vi "WriteCSV.vi"(9 "array":dbl[](array[numeric])=[1.12, 3.14, 0.0], 11 "file path (use dialog)":path=path "C:/Users/RoboIme/git/sslview/Util/Farias2.csv") -> ()   [LabVIEW 2018]
panel:
  out "refnum out":refnum<file>
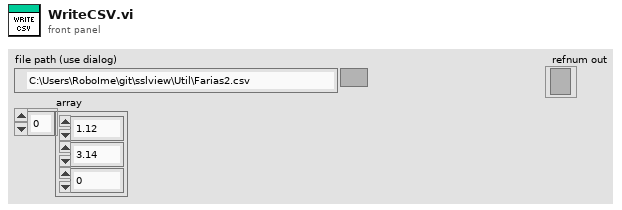
[diagram p1: front panel]
types:
  T1 = enum16{"open", "replace", "create", "open or create", "replace or create", "replace or create with confirmation"}
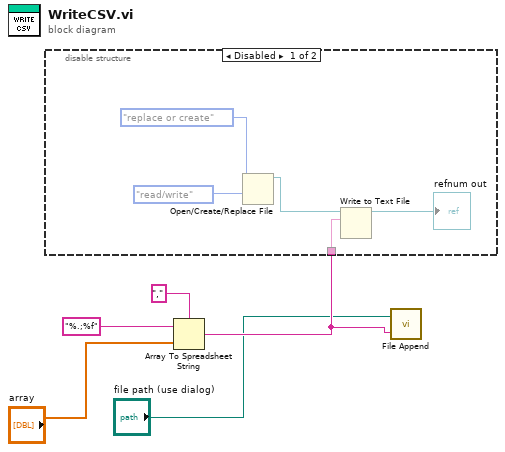
[diagram p0: block diagram]
diagram:
  n1 = Array To Spreadsheet String(delimiter (Tab)=",", array="array", 3:"%.;%f" ("format string")) -> (spreadsheet string=w2:string)
  n2 = disable-structure shown="Disabled" {
    disable-tunnel: w2 -> [w10 _]
    frame Disabled {
      n3 = Open/Create/Replace File(operation (0:open)=T1."replace or create", access (0:read/write)=enum16{"read/write", "read-only", "write-only"}."read/write") -> (refnum out=w7:refnum<file>)  [unwired: 4 in, 2 out]
      n4 = Write to Text File(file (use dialog)=w7, text=w10) -> (refnum out=→"refnum out":refnum<file>)  [unwired: 2 in, 2 out]
    }
    frame Enabled {
    }
  }
  n5 = call "File Append.vi"("string"=w2, "file path"="file path (use dialog)") -> ()  [unwired: 2 in]
